vi "Vision Research Phantom Series PhCon PhGetResolution.vi"(0 "CN in":u32, 2 "pCnt":i32=16, 3 "pCAR":bool, 5 "Error In (no error)":errorcluster) -> (14 "CN out":u32=1, 15 "CAR":T1[](array[typedef]), 16 "pCnt out":i32, 17 "pCar out":bool, 18 "pADCBits":u32, 19 "Error Out":errorcluster)   [LabVIEW 2013, in "VRI.lvlib"]
doc: "PhCon.dll\n\nPhGetResolutions\nHRESULT PhGetResolutions(UINT CN, PPOINT pRes, PUINT pCnt, PBOOL pCAR, PUINT pPixDepth);\n\nParameters Description\nCN (in) Camera number.\npRes (out) Size of the array at input, count of resolutions at output.\npCnt (in, out) If you request one resolution (*pCnt==1 at input) you will get the maximum resolution \n of the camera (512x512 for v4 and 1024x1024 for v5, 800x600 for v7 …).\n pCAR (in, out) -at input\n if pCAR is NULL the result in pRes will be a list of usual resolutions even if the camera \n supports Continuous Adjustable Resolution (CAR)\n -at output, if pCAR is not NULL:\n *pCAR will be TRUE if this camera supports CAR.\n In this case the results in pRes are:\n 0 : Maximum Resolution (compatible with the old style)\n 1 : Minimum Resolution\n 2 : Increments.\n The possible resolutions of a CAR camera are\n X = MinX+i*IncX; i=0...M\n Y = MinY+j*IncY; j=0...N\n where:\n MaxX=pRes[0].x\n MaxY=pRes[0].y\n MinX=pRes[1].x\n MinY=pRes[1].y\n IncX=pRes[2].x\n IncY=pRes[2].y\n M=(MaxX-MinX) / IncX and\n N=(MaxY-MinY) / IncY\n pADCBits (out) Pointer to the maximum bit depth of the pixel values in the camera. \n This is the resolution of the analog to digital converters used for the video digitizing. \nReturn HRESULT (0=Ok)\nComments Get an array with the image dimensions available from this camera and the pixel \n depth. Any pointer can be NULL if that information is not needed but pRes or pCnt \n can be NULL only if both are NULL.\n\nWritten by:\nBLOOMY CONTROLS, INC\nWINDSOR, CT 06095, USA\n860-298-9925\nwww.bloomy.com\nV1.0.0\nMay, 2004"
uses:
  VRI.lvlib
  _Type Defs/Point.ctl
  Phantom DLLs/PhCon.dll
panel:
  out "Raw pRes":u32[](array[numeric])
  # "For instructions on the use of this VI, press Ctrl+H to display the help window and move the mouse over the icon, controls, and indicators"
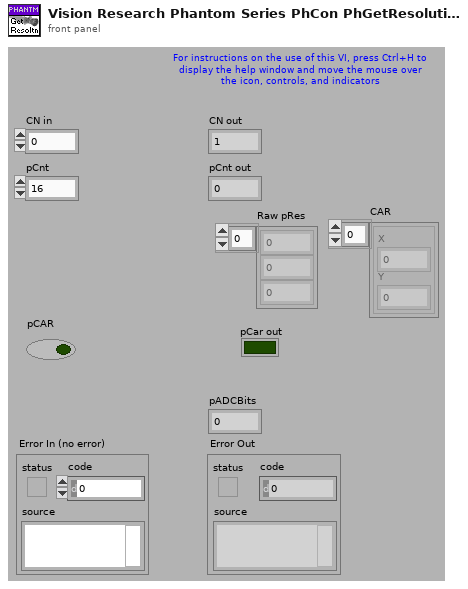
[diagram p1: front panel]
types:
  T1 = typedef "VRI.lvlib/Point.ctl" = cluster{"X":i32, "Y":i32}
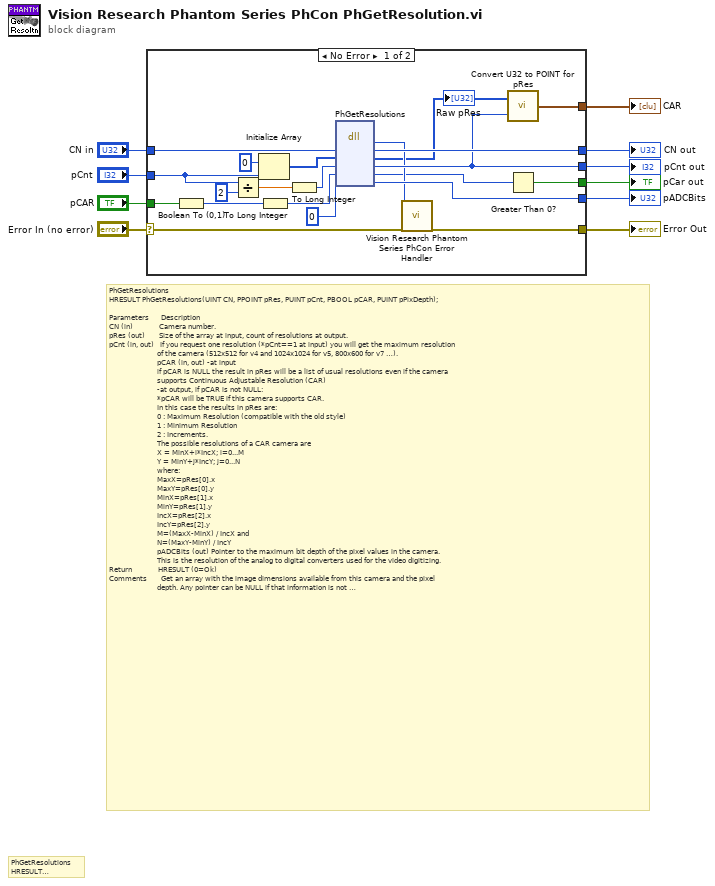
[diagram p0: block diagram]
diagram:
  # "PhGetResolutions\nHRESULT PhGetResolutions(UINT CN, PPOINT pRes, PUINT pCnt, PBOOL pCAR, PUINT pPixDepth);\n\nParameters      Description\nCN (in)             Camera number.\npRes (out)       Size of the array at input, count of resolutions at output.\npCnt (in, out)   If you request one resolution (*pCnt==1 at input) you will get the maximum resolution \n                        of the camera (512x512 for v4 and 1024x1024 for v5, 800x600 for v7 …).\n                        pCAR (in, out) -at input\n                        if pCAR is NULL the result in pRes will be a list of usual resolutions even if the camera \n                        supports Continuous Adjustable Resolution (CAR)\n                        -at output, if pCAR is not NULL:\n                        *pCAR will be TRUE if this camera supports CAR.\n                        In this case the results in pRes are:\n                        0 : Maximum Resolution (compatible with the old style)\n                        1 : Minimum Resolution\n                        2 : Increments.\n                        The possible resolutions of a CAR camera are\n                        X = MinX+i*IncX; i=0...M\n                        Y = MinY+j*IncY; j=0...N\n                        where:\n                        MaxX=pRes[0].x\n                        MaxY=pRes[0].y\n                        MinX=pRes[1].x\n                        MinY=pRes[1].y\n                        IncX=pRes[2].x\n                        IncY=pRes[2].y\n                        M=(MaxX-MinX) / IncX and\n                        N=(MaxY-MinY) / IncY\n                        pADCBits (out) Pointer to the maximum bit depth of the pixel values in the camera. \n                        This is the resolution of the analog to digital converters used for the video digitizing. \nReturn             HRESULT (0=Ok)\nComments       Get an array with the image dimensions available from this camera and the pixel \n                        depth. Any pointer can be NULL if that information is not needed but pRes or pCnt \n                        can be NULL only if both are NULL."
  # "PhGetResolutions\nHRESULT PhGetResolutions(UINT CN, PPOINT pRes, PUINT pCnt, PBOOL pCAR, PUINT pPixDepth);\nParameters Description \nCN (in) Camera number.\npRes (out) Pointer to an array of POINTs with the resolutions.\npCnt (in, out) Size of the array at input, count of resolutions at output.\nIf you request one resolution (*pCnt==1 at input) you will get the maximum resolution of the camera (512x512 for v4 and 1024x1024 for v5, 800x600 for v7 …).\npCAR (in, out) \n-at input, if pCAR is NULL the result in pRes will be a list of usual resolutions even if the camera supports Continuous Adjustable Resolution (CAR)\n-at output, if pCAR is not NULL:\n*pCAR will be TRUE if this camera supports CAR.\nIn this case the results in pRes are:\n0 : Maximum Resolution (compatible with the old style)\n1 : Minimum Resolution\n2 : Increments.\nThe possible resolutions of a CAR camera are\nX = MinX+i*IncX; i=0...M\nY = MinY+j*IncY; j=0...N\nwhere:\nMaxX=pRes[0].x\nMaxY=pRes[0].y\nMinX=pRes[1].x\nMinY=pRes[1].y\nIncX=pRes[2].x\nIncY=pRes[2].y\nM=(MaxX-MinX) / IncX and\nN=(MaxY-MinY) / IncY\npPixDepth (out) effective pixel depth (v4-v6: 8 , v7: 12) on gray images\nReturn HRESULT (0=Ok)\nComments Get an array with the image dimensions available from this camera and the pixel depth.\nAny pointer can be NULL if that information is not needed but pRes or pCnt can be NULL only if both are NULL."
  n1 = case shown="No Error" "Error In (no error)" {
    selector: "Error In (no error)" -> [w31 w35]
    tunnel: [w30 w35] -> w9
    tunnel: "CN in" -> [w29 w34]
    tunnel: [w28 w34] -> w7
    tunnel: [w27 _] -> w6
    tunnel: [w26 w33] -> w5
    tunnel: "pCnt" -> [w25 w33]
    tunnel: "pCAR" -> [w24 w32]
    tunnel: [w23 w32] -> w2
    tunnel: [w22 _] -> w3
    frame No Error {
      n2 = Boolean To (0,1)(Boolean=w24) -> (0, 1=w13:i16)
      n3 = Divide(x=w25, y=2) -> (x/y=w17:dbl)
      n4 = Initialize Array(u32 0 ("Y"), w25) -> (w20:u32[])
      n5 = To Long Integer(number=w13) -> (32bit integer=w12:i32)
      n6 = To Long Integer(number=w17) -> (32bit integer=w16:i32)
      n7 = dll-call lib="C:/Projects/SDK/32-bit/Vision Research Phantom Series Labview Driver/Phantom DLLs/PhCon.dll" fn="PhGetResolutions"("CN"=w29, "pRes"=w20, "pCnt"=w16, "pCAR"=w12, "pADCBits"=u32 0 ("pPixDepth")) -> ("HRESULT"=w21:i32, "CN"=w28:u32, "pRes"=w15:u32[], "pCnt"=w26:i32, "pCAR"=w14:i32, "pADCBits"=w27:u32)  [unwired: 3 in, 2 out]
      "Raw pRes" <- w15
      n8 = call "Vision Research Phantom Series PhCon Error Handler.vi"("ErrNo"=w21, "Error In (no error)"=w31) -> ("Error Out"=w30:errorcluster)  [unwired: 17 out]
      n9 = call "Convert U32 to POINT for pRes.vi"("pCnt"=w26, "pRes 2"=w15) -> ("pRes"=w22:T1[])
      n10 = Greater Than 0?(x=w14) -> (x > 0?=w23:bool)
    }
    frame Error {
    }
  }
  "Error Out" <- w9
  "CN out" <- w7
  "pADCBits" <- w6
  "pCnt out" <- w5
  "CAR" <- w3
  "pCar out" <- w2
